vi "start digital software pulse .vi"(9 "frequency":i32, 10 "pin":i32, 11 "handle":u32) -> (2 "function return":bool, 3 "handle out":u32)   [LabVIEW 2020, in "cDaq.lvlib"]
doc: "DAQAPI bool start_digital_software_pulse_(HDAQ handle, int pin, int frequency);"
uses:
  cDaq.lvlib
  cDaq.dll
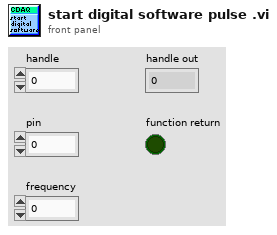
[diagram p1: front panel]
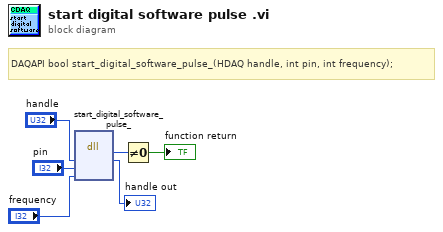
[diagram p0: block diagram]
diagram:
  # "DAQAPI bool start_digital_software_pulse_(HDAQ handle, int pin, int frequency);"
  n1 = dll-call lib="G:/CODE/01-Cplusplus/cDaq/doc/UsingWithLabview/cDaqlib/cDaq.*" fn="start_digital_software_pulse_"("handle"="handle", "pin"="pin", "frequency"="frequency") -> (w5:u8, "handle"=→"handle out":u32)  [unwired: 5 in, 2 out]
  n2 = Not Equal To 0?(x=w5) -> (x != 0?=→"function return":bool)
